vi "Master Setup Subpanel.vi"() -> ()   [LabVIEW 2017]
uses:
  Setup File Operations/File Operation with History Buttons.ctl
  Master Setup Export to Compressed Zip Folder.ctl
  Master Setup Import to Compressed Zip Folder.ctl
  Master Setup Open Backup Scheduler.ctl
  Setup File Operations/File Operation with History.ctl
  Master Setup States Enum.ctl
  <vilib>/Utility/miscctls.llb/LVRowAndColumnTypeDef.ctl
  Master Setup Pattern Enum.ctl
  <vilib>/Utility/config.llb/NI_LVConfig.lvlib
panel:
  in  "Backup Scheduler":T1
  in  "Tab Control":T2(tab)
  in  "Master Setup File List":i32(listbox)=-1
  out "Master Save Status":bool[](array[boolean])
  out "Master Open Status":bool[](array[boolean])
  out "Master Setup Titles":string[](array[string])=["0 - Channel Setup", "1 - PID Setup", "2 - Filter Setup", "3 - CAN Message Setup", "4 - CAN 1 Setup", "5 - CAN 2 Setup", "6 - Digital Inputs Setup", "7 - Digital Outputs Setup", "8 - Logging 1 Setup", "9 - Logging 2 Setup", "10 - Logging 3 Setup", "11 - Setpoint Setup", "12 - Test Series Setup", "13 - Graph Setup", "14 - System Configure", "15 - Header", "16 - Profile Manager", "17 - Post-Mortem Logging", "18 - High-Speed Data", "19 - Statistic Channel Setup", "20 - Ramp Channel Setup", "21 - ETAS INCA Channel Setup", "22 - ETC ECCS Transducer Setup", "23 - ETC ECCS Test Setup", "24 - AVL AK Smoke Meter Setup", "25 - Triggers Setup", "26 - Alarm Limits Setup", "27 - YKWT1 Measurement", "28 - YKWT1 Instrument", "29 - Auto File Settings", "30 - Playback File Setting", "31 - UUT Constants", "32 - UPS Setup", "33 - Differential Channel Setup", "34 - Integral Channel Setup", "35 - Signal Channel Setup", "36 - Calibration Setup", "37 - BNC Setup", "38 - ASAP3 Setup", "39 - Chassis Force Calculations", "40 - Chassis Teststand Losses", "41 - Chassis Vehicle Losses", "42 - Formula Channels", "43 - ASAP3 Map Coords Setup", "44 - Digital Controls Setup", "45 - Push Buttons Setup", "46 - Sliders Setup", "47 - Analog Inline Filter Setup", "48 - Email Setup", "49 - Timer Setup", "50 - Unit Conversion Setup", "51 - Visible Channels", "52 - Main Display Setup", "53 - Message Display Setup", "54 - Input Display Setup", "55 - Unico Parameter Downloads", "56 - Flow Meter Setup", "57 - Channel Zero Offset", "58 - YKWT2 Measurement", "59 - YKWT2 Instrument", "60 - CAN 3 Setup", "61 - CAS Setup", "62 - Accumulation Channel Setup", "63 - Valvetrain Dynamics Setup", "64 - CCP Setup", "65 - System Log Setup", "66 - Throttle Controller", "67 - RE Shifter", "68 - Main Display"]
  out "File Error":bool[](array[boolean])
  out "Convert Error":bool[](array[boolean])
  out "RT Update Error":bool[](array[boolean])
  in  "Refresh":bool
  in  "Master Open":bool
  in  "Master Save":bool
  in  "Master Exit":bool
  out "Login User":string
  out "Progress":i32(slide) scale=0.0..73.0
  out "File Path":path
  out "Last Time Saved":timestamp
  out "Master Open Indicator":bool
  out "Master Save Indicator":bool
  in  "WinZIP Import":T3
  in  "WinZIP Export":T4
  in  "File Operations with History Buttons":T5
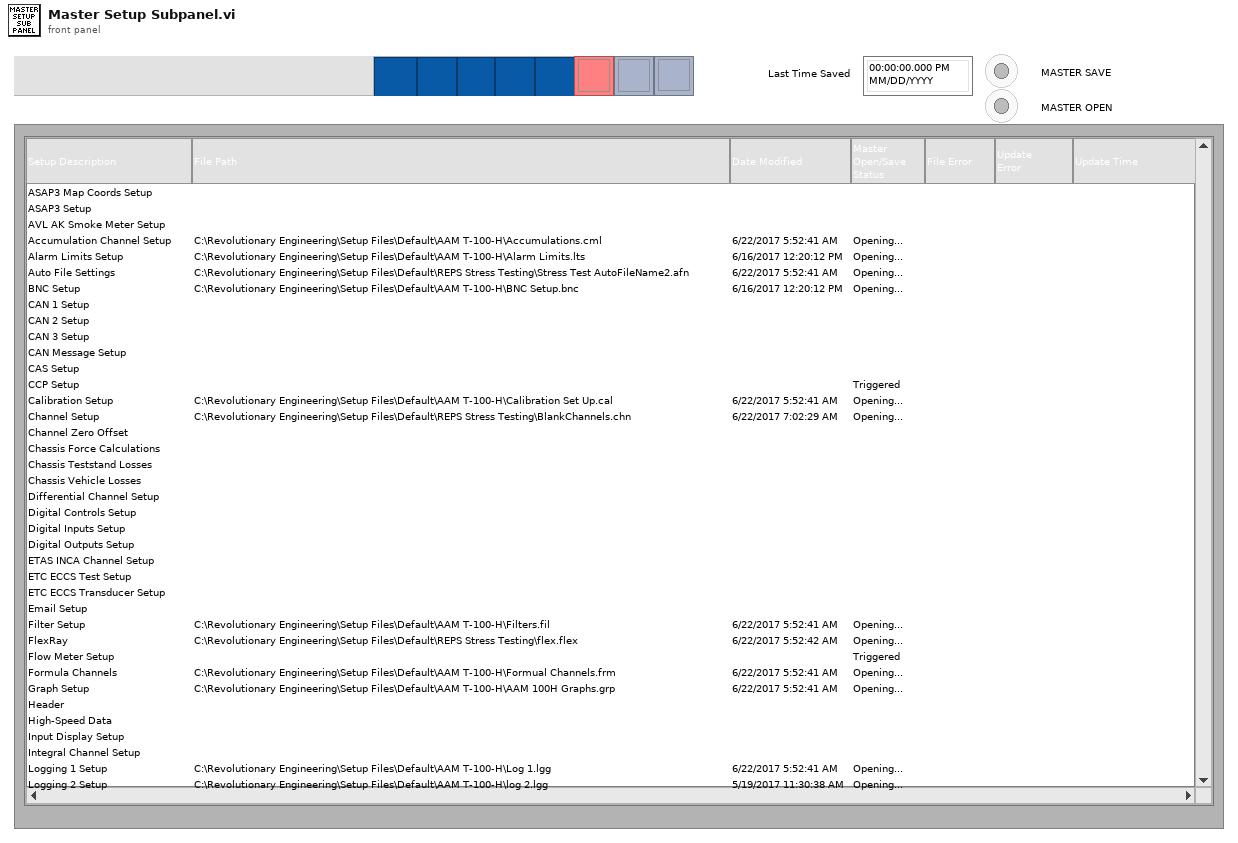
[diagram p1: front panel]
types:
  T1 = typedef "Master Setup Open Backup Scheduler.ctl" = bool
  T2 = enum32{"Master Setup List", "Master Setup Status", "File Update Event Log "}
  T3 = typedef "Master Setup Import to Compressed Zip Folder.ctl" = bool
  T4 = typedef "Master Setup Export to Compressed Zip Folder.ctl" = bool
  T5 = typedef "File Operation with History Buttons.ctl" = cluster{"New":bool, "Browse - Open":bool, "Save":bool, "Save As":bool, "Recent Files - Open":bool}
  T6 = typedef "Master Setup States Enum.ctl" = enum16{"Initialize", "Update Display", "Poll", "Prompt to Save", "Master Save", "Master Open", "Open Recent Dialog", "Open Normal Dialog", "Open Selected Master File", "WINZIP Export", "WINZIP Import", "WINZIP Auto Backup", "Exit"}
  T7 = typedef "File Operation with History.ctl" = cluster{"Operator New":bool, "Operator Open":bool, "Operator Save":bool, "Operator Save As":bool, "Master Open":bool, "Master Save":bool, "Shortcut Open (From Menu)":bool, "Shortcut Open (From Button)":bool}
  T8 = cluster{"Sorted Titles Indices":i32[], "Sorted Titles":string[], "Master Setup Path":path, "Master Setup Table":string[][], "First Run":bool, "Master Pattern":string, "Master Pattern Label":string, "Skip Save Prompt?":bool}
  T9 = typedef "LVRowAndColumnTypeDef.ctl" = cluster{"Row":i32, "Column":i32}
  T10 = enum16{"Read String Queue", "Write String Queue", "Read U16 Queue", "Write U16 Queue"}
  T11 = enum32{"Invalid", "Standard", "Closed", "Hidden", "Minimized", "Maximized"}
  T12 = enum16{"Get Master Open Status", "Get Master Save Status"}
  T13 = enum16{"open", "replace", "create", "open or create", "replace or create", "replace or create with confirmation"}
  T14 = typedef "PC_INI_Data__TypeDef.ctl" = cluster{"REPS Version":T15, "System Configuration":T16, "OPC PLC Write":string, "OPC PLC Read":string, "Modbus Info":string, "INCA Configuration":cluster{"IP":string, "Port":i32, "Protocol Version":i32}, "ECCS Setup":cluster{"Enable":bool, "IP":string, "TCP Port":u16, "UDP Port":u16, "Engine ODBC Name":string, "Fuel ODBC Name":string}, "Encoder Configuration":cluster{"Encoder1PPR":i32, "Encoder1Interval1":i32, "Encoder1Interval2":i32, "Roll Diameter(Feet)":i32, "Encoder2PPR":i32, "Encoder3PPR":i32, "Encoder4PPR":i32, "Encoder5PPR":i32, "Encoder2Interval1":i32, "Encoder2Interval2":i32, "Encoder3Interval1":i32, "Encoder3Interval2":i32}, "Pickup1 Configuration":cluster{"PickupPPR":i32, "PickupInterval1":i32, "PickupInterval2":i32}, "Pickup2 Configuration":cluster{"PickupPPR":i32, "PickupInterval1":i32, "PickupInterval2":i32}, "Pickup3 Configuration":cluster{"PickupPPR":i32, "PickupInterval1":i32, "PickupInterval2":i32}, "Shifter Configuration":cluster{"RE Shifter Enable":bool, "Shifter IP Address":string, "Shifter Port":u16}, "Misc Configuration":T17, "Logging Configuration":T18}
  T15 = typedef "REPS Version.ctl" = cluster{"Version":string}
  T16 = typedef "System Configuration.ctl" = cluster{"Cell":string, "DualMotorSet":bool, "Hardware Setup Array":bool[], "Host IP":string, "Remote IP 1":string, "Remote IP 2":string, "Remote IP 3":string, "Remote Enable 1":bool, "Remote Enable 2":bool, "Remote Enable 3":bool, "Company Name":string, "Company Info":string, "Number Of Modbus":i32, "Setup Files Path":path, "Master File Path":path, "Master Setup Titles":string[], "Encoder1PPR":i32, "Encoder1Interval1":i32, "Encoder1Interval2":i32, "Display File Error Status?":bool[], "Update to RT Delay":u32, "Formula Rate (Hz)":u32, "Custom Screen (Left) Path":path, "Custom Screen (Right) Path":path}
  T17 = typedef "Misc Configuration.ctl" = cluster{"Show PM Logging Indicator":bool}
  T18 = typedef "Logging Configuration.ctl" = cluster{"MaxLogFileSize":T19, "MaxNumofLogChannels":T19, "MaxNumofPMLogChannels":T19, "SkipPMDialog":i32}
  T19 = typedef "Framed Numeric 6 digit 20 point.ctl" = dbl
  T20 = typedef "NI_LVConfig.lvlib/Config Data RefNum.ctl" = refnum<k1>
  T21 = typedef "Master Setup Pattern Enum.ctl" = i32
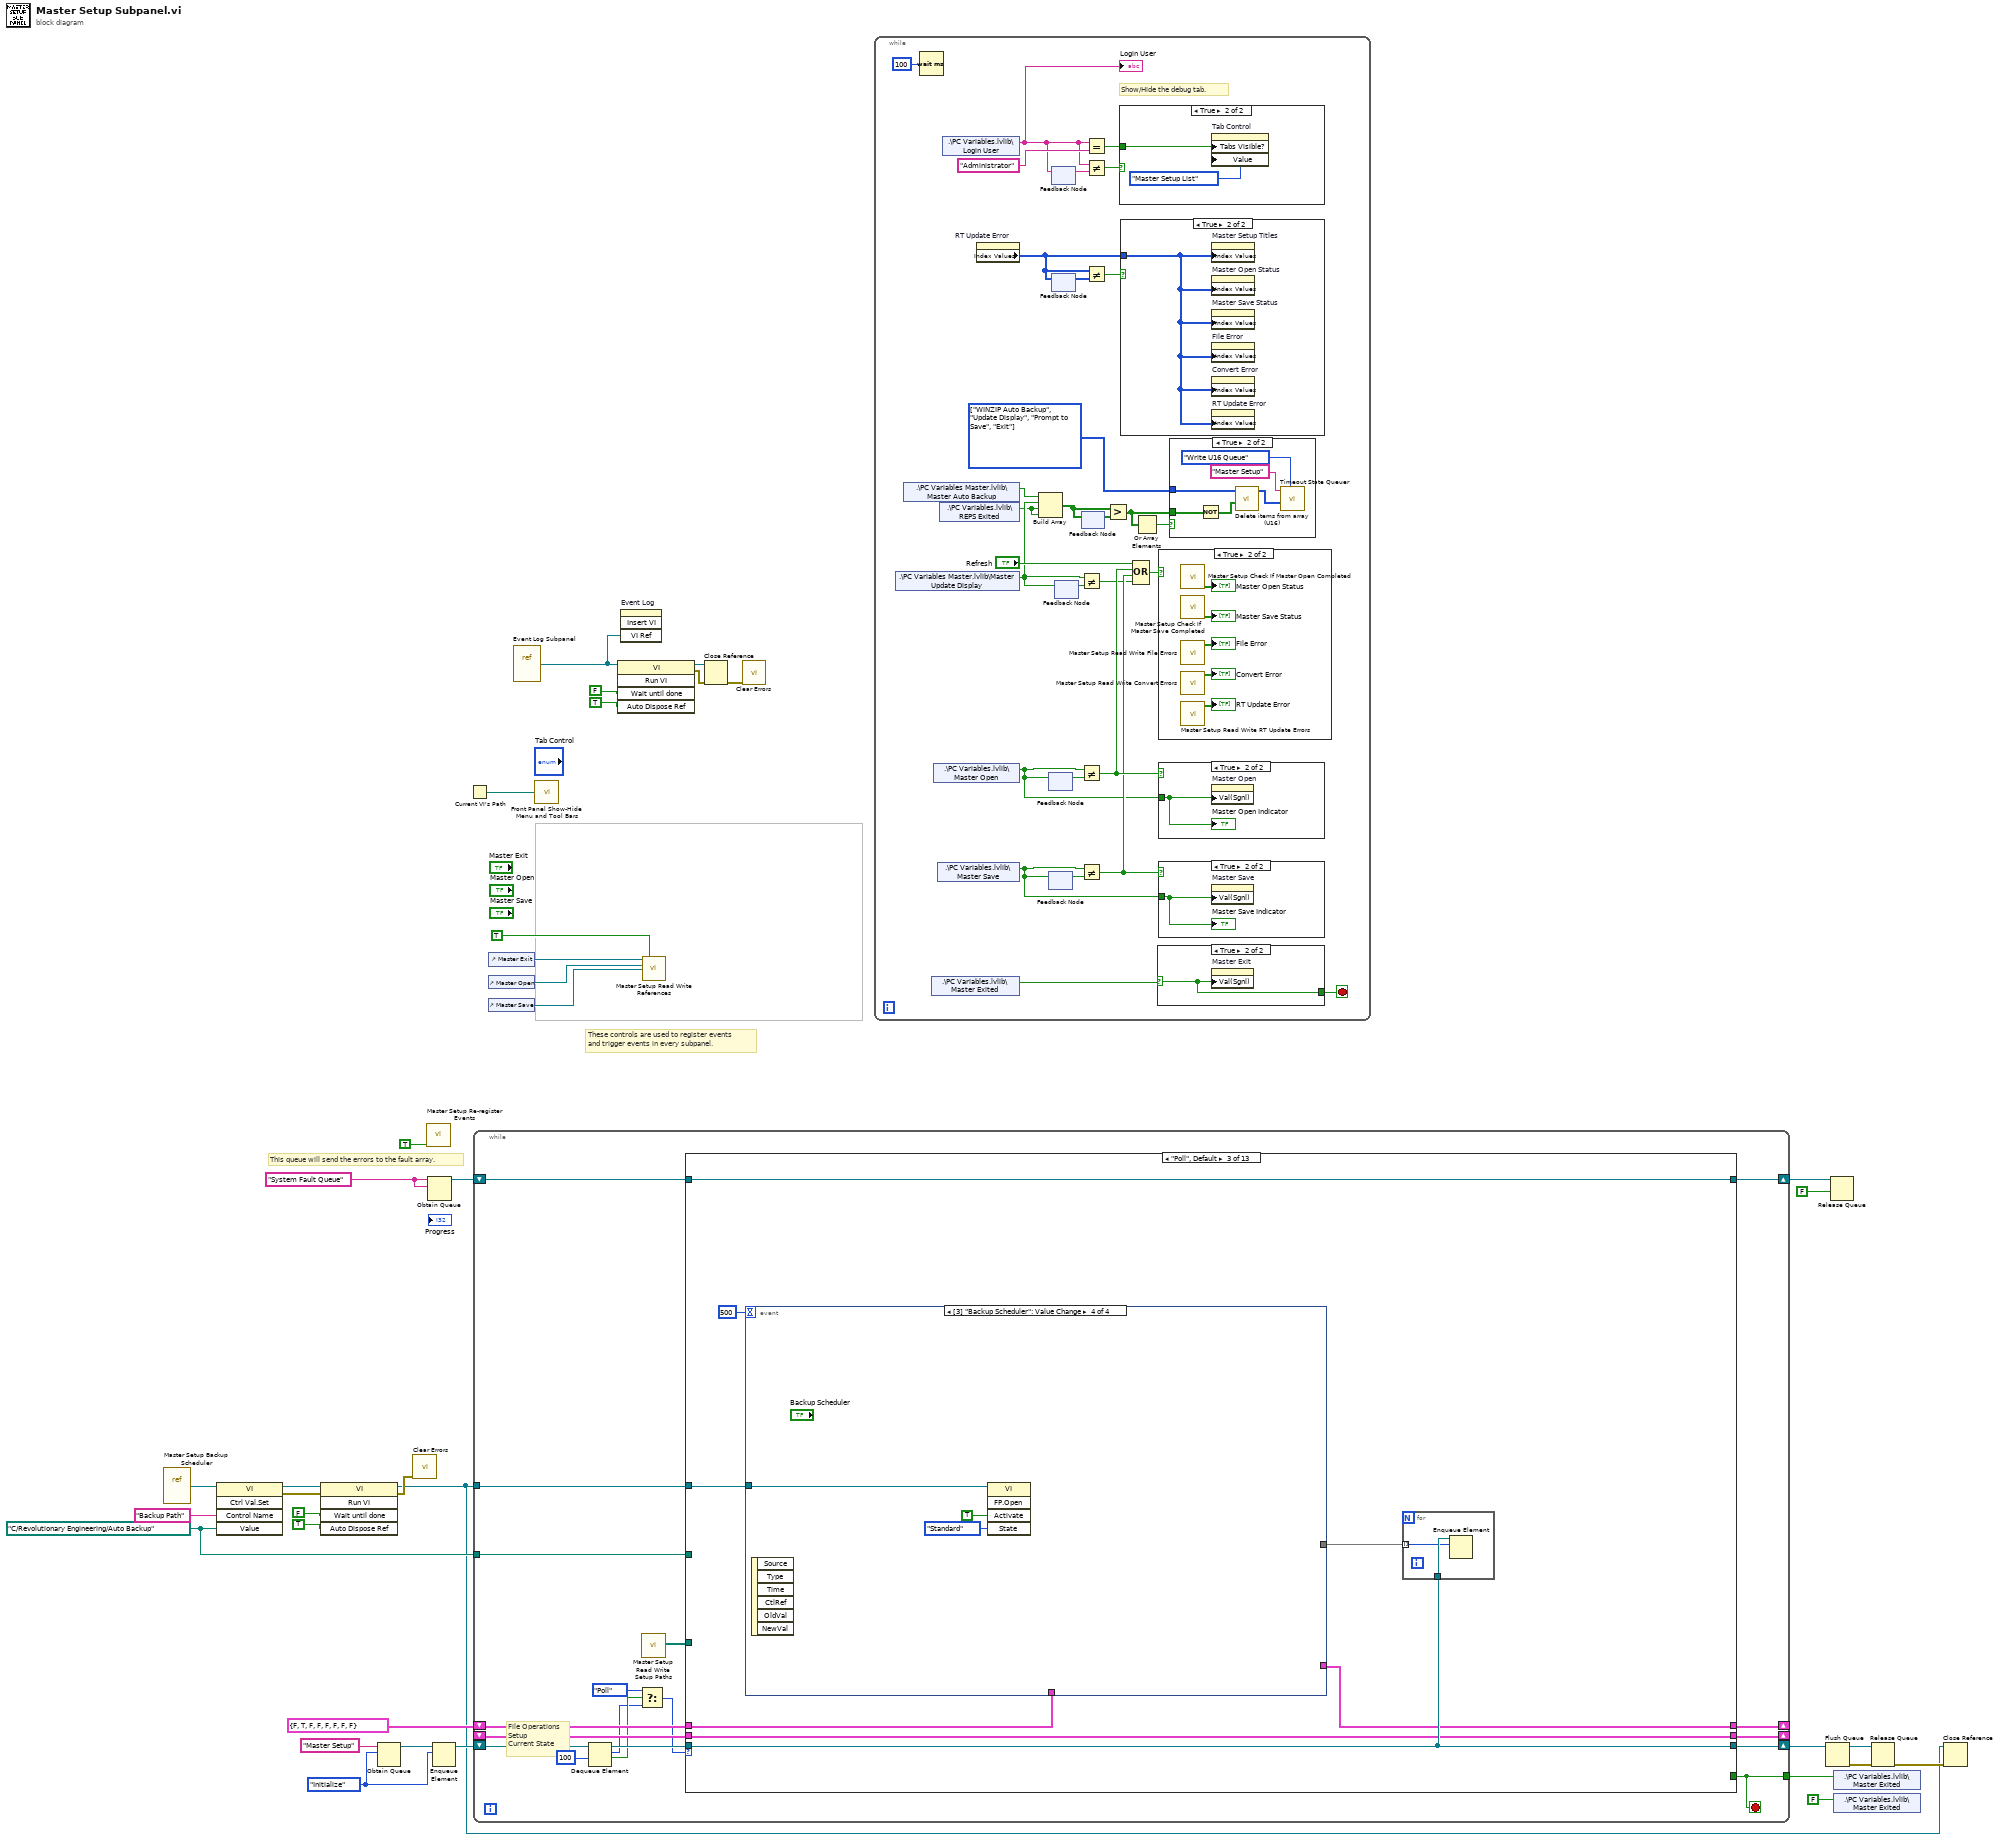
[diagram p0: block diagram]
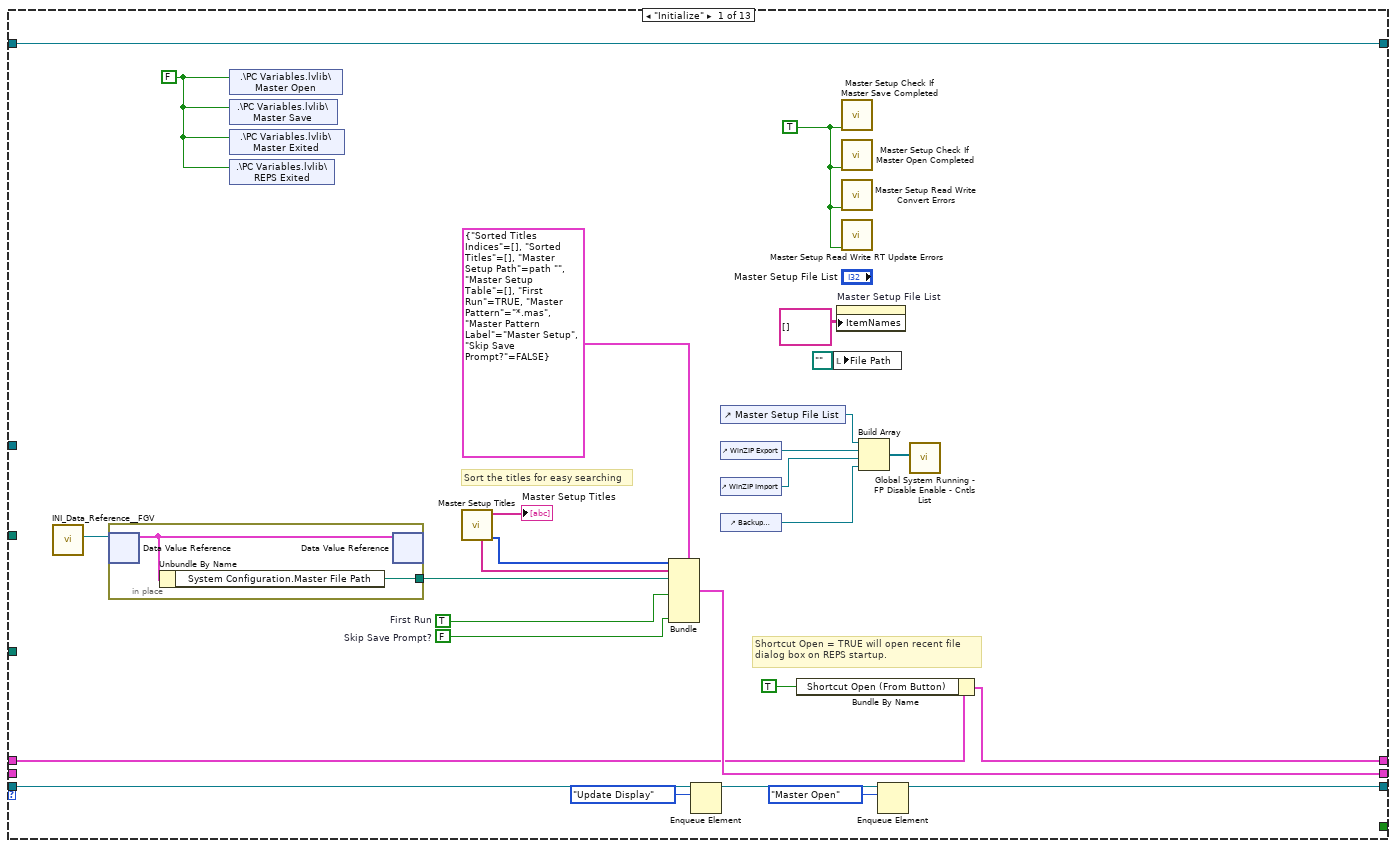
[diagram p9: hidden frame]
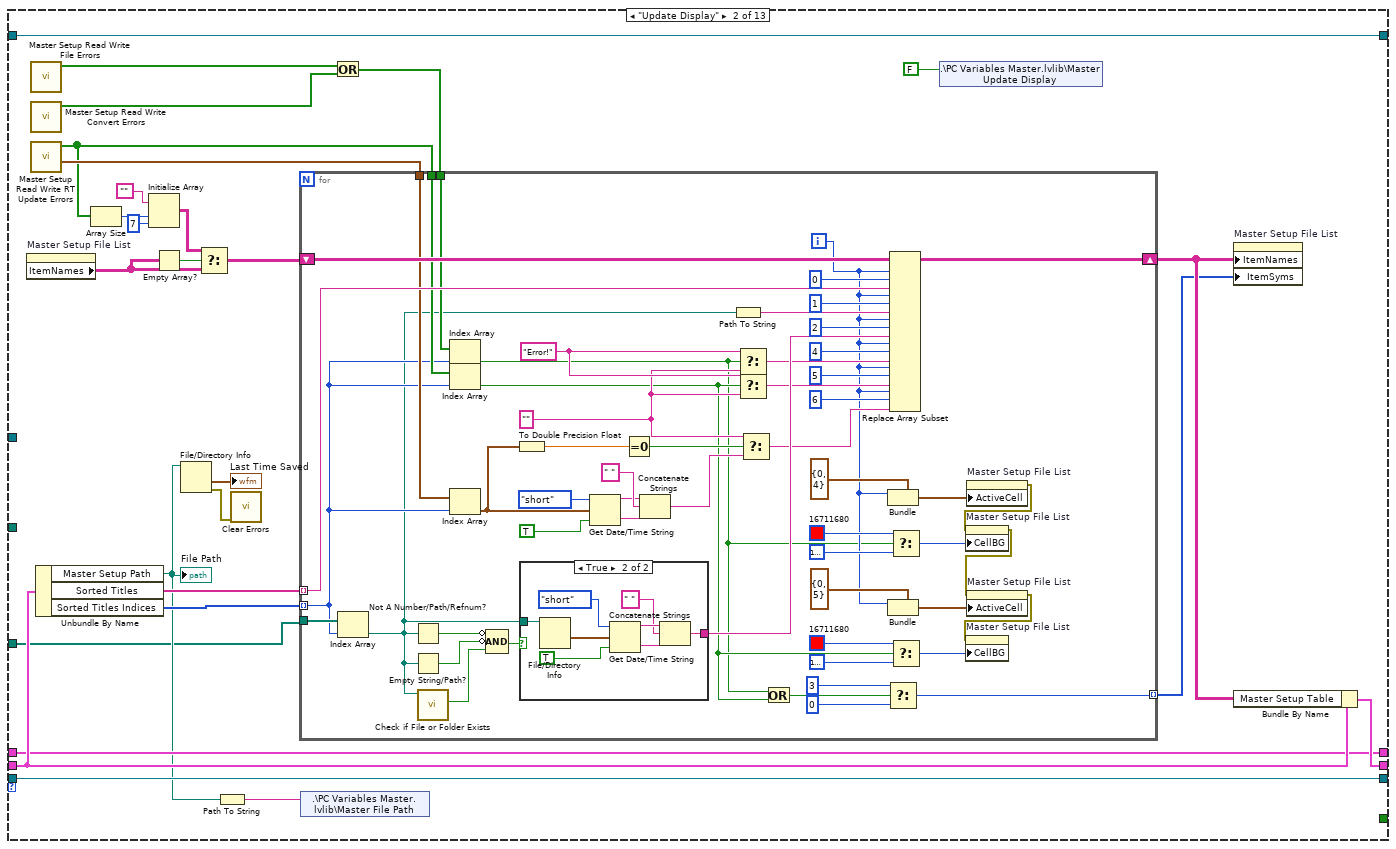
[diagram p10: hidden frame]
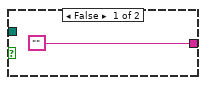
[diagram p11: hidden frame]
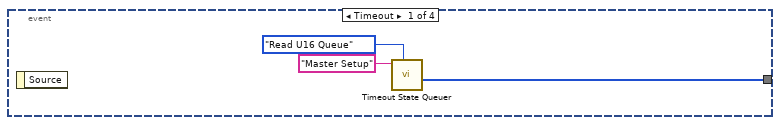
[diagram p12: hidden frame]
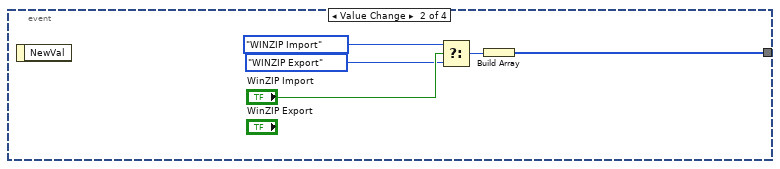
[diagram p13: hidden frame]
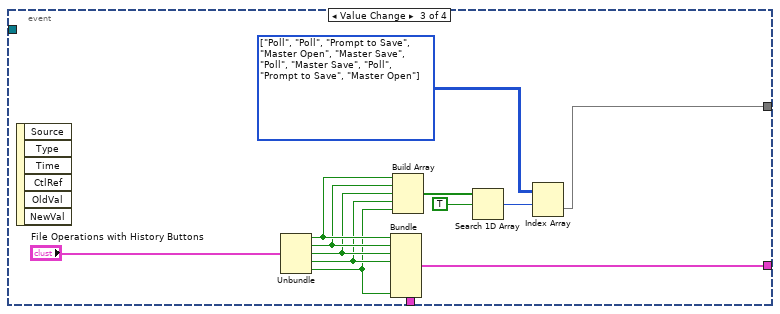
[diagram p14: hidden frame]
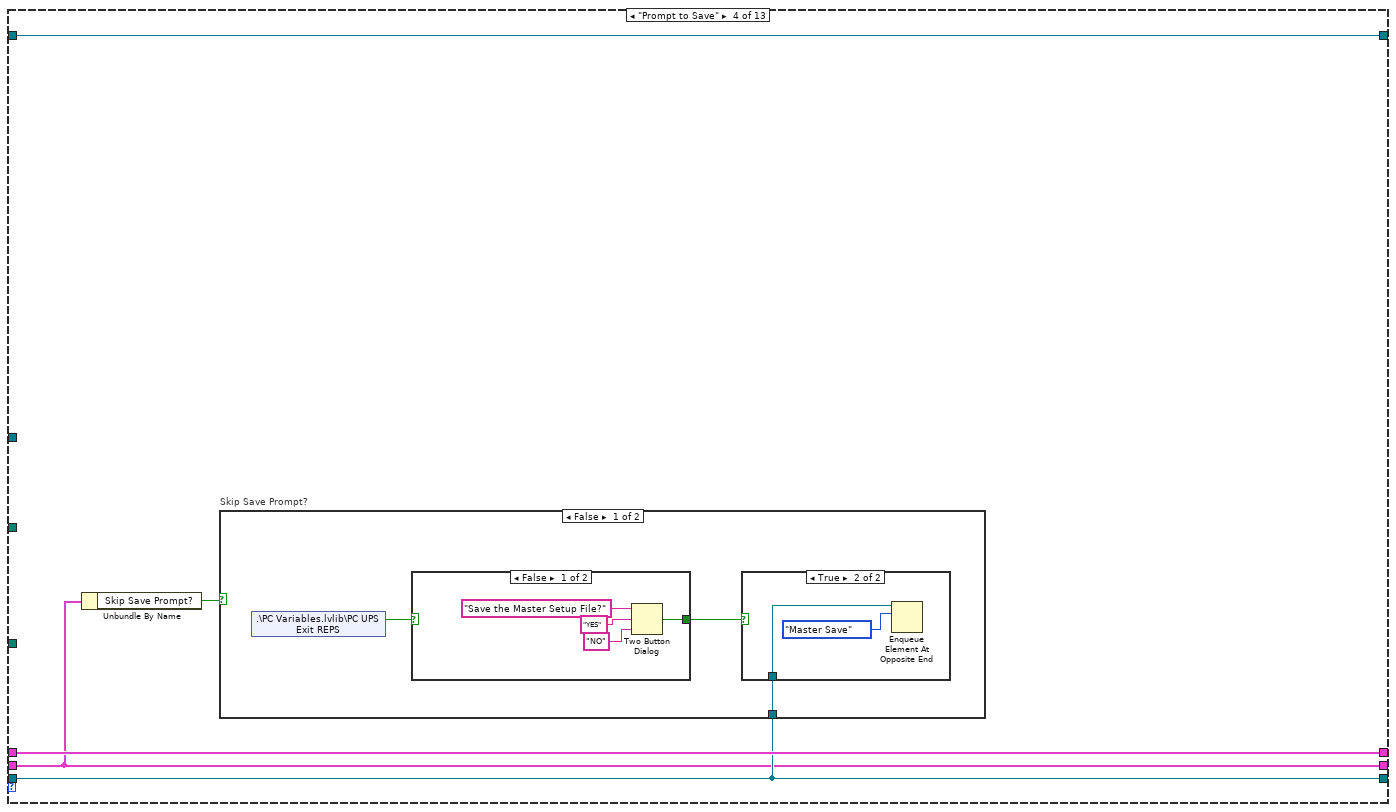
[diagram p15: hidden frame]
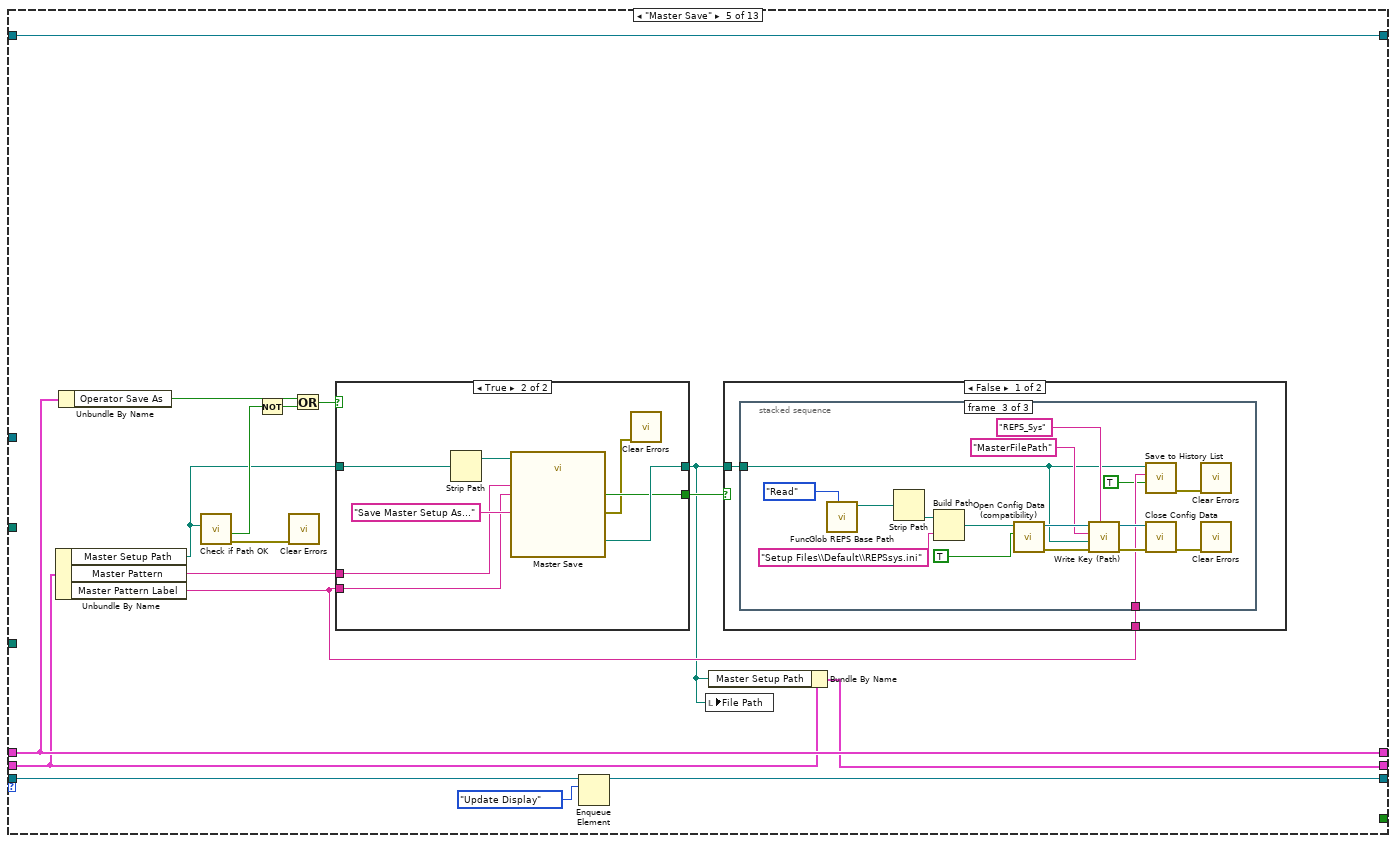
[diagram p19: hidden frame]
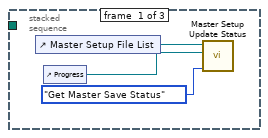
[diagram p20: hidden frame]
diagram:
  w5 = path "C:/Revolutionary Engineering/Auto Backup"
  w13 = Master_Setup_States_Enum."Initialize" ("States")
  w24 = "System Fault Queue" ("name (unnamed)")
  # "These controls are used to register events \nand trigger events in every subpanel."
  # "This queue will send the errors to the fault array."
  n1 = vi-ref "Master Setup Backup Scheduler.vi"() -> (w11:refnum<vi>)
  n2 = invoke class="VI" method="Ctrl Val.Set"(reference=w11, "Control Name"="Backup Path", "Value"=w5) -> (reference out=w8:refnum<vi>, error out=w9:errorcluster)  [unwired: 2 in, 3 out]
  n3 = invoke class="VI" method="Run VI"(reference=w8, error in=w9, "Wait until done"=FALSE ("Wait Until Done"), "Auto Dispose Ref"=TRUE ("Auto Dispose Reference")) -> (reference out=w3:refnum<vi>, error out=w12:errorcluster)  [unwired: 1 in, 3 out]
  n4 = Obtain Queue(name (unnamed)="Master Setup", element data type=w13) -> (queue out=w15:refnum<queue>)  [unwired: 3 in, 2 out]
  n5 = call <vilib>:"Clear Errors.vi"("error in (no error)"=w12) -> ()  [unwired: 5 in, 2 out]
  n6 = call "Master Setup Re-register Events.vi"("Master/Channel Subpanel Restarted"=TRUE) -> ()  [unwired: 10 in, 1 out]
  n7 = Obtain Queue(name (unnamed)=w24, element data type=w24) -> (queue out=w27:refnum<queue>)  [unwired: 3 in, 2 out]
  n8 = Enqueue Element(queue=w15, element=w13) -> (queue out=w14:refnum<queue>)  [unwired: 2 in, 2 out]
  n9 = Current VI's Path() -> (path=w22:path)
  n10 = while {
    shift-right: [w52] -> w32
    shift-left: w14 -> [w44]
    shift-right: [w51] -> _
    shift-left: _ -> [w54]
    shift-right: [w49] -> _
    shift-left: T7 {"Operator New"=FALSE, "Operator Open"=TRUE, "Operator Save"=FALSE, "Operator Save As"=FALSE, "Master Open"=FALSE, "Master Save"=FALSE, "Shortcut Open (From Menu)"=FALSE, "Shortcut Open (From Button)"=FALSE} ("File Operation (in)") -> [w48]
    tunnel: [w47] -> w1
    shift-right: [w45] -> w26
    shift-left: w27 -> [w46]
    tunnel: w5 -> [w38]
    tunnel: w3 -> [w37]
    stop <- w47 stop-if-true
    # "File Operations\nSetup\nCurrent State"
    n11 = Dequeue Element(queue=w44, timeout in ms (-1)=100) -> (queue out=w53:refnum<queue>, element=w42:T6, timed out?=w43:bool)  [unwired: 1 in, 1 out]
    n12 = Select(t=Master_Setup_States_Enum."Poll", s=w43, f=w42) -> (s? t:f=w40:T6)
    n13 = call "Master Setup Read Write Setup Paths.vi"() -> ("New Setup Paths"=w39:path[])  [unwired: 7 in, 4 out]
    n14 = case shown="\"Poll\", Default" w40 {
      tunnel: w54 -> [_ w95 w176 w210 w226 w283 w393 w439 w471 w494 w509 w533 w555]
      tunnel: w53 -> [w68 w110 w181 w211 w231 w285 w389 w442 w480 w495 w511 w549 w554]
      tunnel: [w75 w110 w181 w211 w230 w288 w388 w441 w480 w495 w505 w549 w554] -> w52
      tunnel: [w81 w107 w176 w210 w225 w284 w392 w438 w472 w494 w508 w533 w555] -> w51
      tunnel: [w64 w94 w179 w212 w227 w286 w399 w443 w479 w496 w512 w548 w556] -> w49
      tunnel: w48 -> [w65 w94 w180 w212 w227 w287 w399 w443 w479 w496 w512 w548 w556]
      tunnel: [_ _ _ _ _ _ _ _ _ _ _ _ TRUE] -> w47
      tunnel: w46 -> [w73 w90 w177 w213 w240 w289 w398 w450 w478 w490 w502 w547 w557]
      tunnel: [w73 w90 w177 w213 w240 w289 w398 w450 w478 w490 w502 w547 w557] -> w45
      tunnel: w39 -> [_ w86 _ _ _ _ _ _ _ w489 w500 w532 _]
      tunnel: w38 -> [_ _ _ _ _ _ _ _ _ _ _ w531 _]
      tunnel: w37 -> [_ _ w175 _ _ _ _ _ _ _ _ _ _]
      frame "Initialize" {
        w62 = FALSE  # Skip Save Prompt?
        w71 = FALSE ("Master Open")
        w74 = TRUE ("Reset")
        w66 = TRUE  # First Run
        # "Shortcut Open = TRUE will open recent file\ndialog box on REPS startup."
        # "Sort the titles for easy searching"
        n15 = call "INI_Data_Reference__FGV.vi"() -> (".ini Data Value Reference (out)"=w56:refnum<data-value>)  [unwired: 11 in]
        n16 = in-place {
          in-place-border: [w82] -> w55
          n17 = in-place-dvr #1(w56) -> (w83:T14)  [unwired: 1 out]
          n18 = Unbundle By Name(w83) -> ("System Configuration.Master File Path"=w82:path)
          n19 = in-place-dvr #1(w83) -> ()  [unwired: 2 out]
        }
        n20 = shared-variable ".\\PC Variables.lvlib\\Master Open"(w71) -> ()  [unwired: 1 in, 1 out]
        n21 = shared-variable ".\\PC Variables.lvlib\\Master Save"(w71) -> ()  [unwired: 1 in, 1 out]
        n22 = shared-variable ".\\PC Variables.lvlib\\Master Exited"(w71) -> ()  [unwired: 1 in, 1 out]
        n23 = shared-variable ".\\PC Variables.lvlib\\REPS Exited"(w71) -> ()  [unwired: 1 in, 1 out]
        n24 = call "Master Setup Titles.vi"() -> ("Sorted Titles Indices"=w76:i32[], "Setup Description w/Numbers"=→"Master Setup Titles":string[], "Sorted Setup Description"=w77:string[])  [unwired: 6 in, 3 out]
        n25 = Bundle(cluster=T8 {"Sorted Titles Indices"=[], "Sorted Titles"=[], "Master Setup Path"=path "", "Master Setup Table"=[], "First Run"=TRUE, "Master Pattern"="*.mas", "Master Pattern Label"="Master Setup", "Skip Save Prompt?"=FALSE}, "Sorted Titles Indices"=w76, "Sorted Titles"=w77, "Master Setup Path"=w55, "First Run"=w66, "Skip Save Prompt?"=w62) -> (w81:T8)  [unwired: 3 in]
        n26 = Enqueue Element(queue=w68, element=Master_Setup_States_Enum."Update Display") -> (queue out=w67:refnum<queue>)  [unwired: 2 in, 2 out]
        n27 = control-ref of="Master Setup File List"() -> (w60:refnum<vi>)
        n28 = control-ref of="WinZIP Export"() -> (w59:refnum<vi>)
        n29 = control-ref of="WinZIP Import"() -> (w58:refnum<vi>)
        n30 = control-ref of="Backup Scheduler"() -> (w57:refnum<vi>)
        n31 = Bundle By Name(cluster=w65, "Shortcut Open (From Button)"=TRUE) -> (w64:T7)
        n32 = local write "File Path"(path "" ("File Path")) -> ()
        n33 = property on="Master Setup File List" class="MCListbox (strict)"("ItemNames"=string[][] [] ("Item Names")) -> ()  [unwired: 2 in, 2 out]
        n34 = call "Master Setup Check If Master Save Completed.vi"("Reset"=w74) -> ()  [unwired: 6 in, 5 out]
        n35 = call "Master Setup Check If Master Open Completed.vi"("Reset"=w74) -> ()  [unwired: 6 in, 5 out]
        n36 = call "Master Setup Read Write Convert Errors.vi"("Reset"=w74) -> ()  [unwired: 9 in, 2 out]
        n37 = call "Master Setup Read Write RT Update Errors.vi"("Reset"=w74) -> ()  [unwired: 8 in, 3 out]
        n38 = Build Array(w60, w59, w58, w57) -> (w61:refnum<vi>[])
        n39 = Enqueue Element(queue=w67, element=Master_Setup_States_Enum."Master Open") -> (queue out=w75:refnum<queue>)  [unwired: 2 in, 2 out]
        n40 = call "Global System Running - FP Disable Enable - Cntls List.vi"("Cntls Should NOT be disabled In[]"=w61) -> ()  [unwired: 8 in, 3 out]
      }
      frame "Update Display" {
        n41 = property on="Master Setup File List" class="MCListbox (strict)"() -> ("ItemNames"=w103:string[][])  [unwired: 2 in, 2 out]
        n42 = call "Master Setup Read Write File Errors.vi"() -> ("File Error (out)"=w93:bool[])  [unwired: 10 in, 1 out]
        n43 = call "Master Setup Read Write Convert Errors.vi"() -> ("Convert Error (out)"=w92:bool[])  [unwired: 10 in, 1 out]
        n44 = call "Master Setup Read Write RT Update Errors.vi"() -> ("Update Timestamp"=w97:timestamp[], "Real-Time Update Status (out)"=w96:bool[])  [unwired: 9 in, 1 out]
        n45 = Unbundle By Name(w95) -> ("Master Setup Path"=w87:path, "Sorted Titles"=w108:string[], "Sorted Titles Indices"=w109:i32[])
        "File Path" <- w87
        n46 = Array Size(array=w96) -> (size(s)=w102:i32)
        n47 = Initialize Array("", w102, 7 ("dimension size")) -> (w99:string[][])
        n48 = Empty Array?(array=w103) -> (empty?=w105:bool)
        n49 = File/Directory Info(path=w87) -> (last mod=→"Last Time Saved":timestamp, error out=w88:errorcluster)  [unwired: 1 in, 5 out]
        n50 = Select(t=w99, s=w105, f=w103) -> (s? t:f=w104:string[][])
        n51 = Path To String(path=w87) -> (string=w84:string)
        n52 = call <vilib>:"Clear Errors.vi"("error in (no error)"=w88) -> ()  [unwired: 5 in, 2 out]
        n53 = shared-variable ".\\PC Variables Master.lvlib\\Master File Path"(w84) -> ()  [unwired: 1 in, 1 out]
        n54 = Or(x=w93, y=w92) -> (x .or. y?=w91:bool[])
        n55 = for {
          tunnel: w86 -> [w162]
          tunnel: w109 -> [w123] mode=indexing
          tunnel: w108 -> [w158] mode=indexing
          tunnel: w91 -> [w124]
          tunnel: w96 -> [w125]
          shift-right: [w159] -> w106
          shift-left: w104 -> [w160]
          tunnel: [w143] -> w98 mode=indexing
          tunnel: w97 -> [w127]
          i -> [w116]
          w128 = ""
          w130 = "Error!" ("Setup Description")
          n56 = Index Array(array=w162, index=w123) -> (element=w111:path)
          n57 = Not A Number/Path/Refnum?(number/path/refnum=w111) -> (NaN/Path/Refnum?=w163:bool)
          n58 = Empty String/Path?(string/path=w111) -> (empty?=w165:bool)
          n59 = call <vilib>:"Check if File or Folder Exists.vi"("path"=w111) -> ("file or folder exists?"=w164:bool)  [unwired: 8 in, 2 out]
          n60 = Index Array(array=w124, index=w123) -> (element=w114:bool)
          n61 = Index Array(array=w125, index=w123) -> (element=w115:bool)
          n62 = Index Array(array=w127, index=w123) -> (element=w126:timestamp)
          n63 = Compound Arithmetic op=AND(invert w163, invert w165, w164) -> (w161:bool)
          n64 = To Double Precision Float(number=w126) -> (double precision float=w137:dbl)
          n65 = case shown="True" w161 {
            tunnel: ["" w174] -> w152
            tunnel: w111 -> [_ w173]
            frame False {
            }
            frame True {
              n66 = File/Directory Info(path=w173) -> (last mod=w172:timestamp)  [unwired: 1 in, 6 out]
              n67 = Get Date/Time String(date format (0)=enum16{"short", "long", "abbreviated"}."short", seconds (now)=w172, want seconds? (F)=TRUE) -> (date string=w170:string, time string=w169:string)
              n68 = Concatenate Strings(w170, " " ("string"), w169) -> (w174:string)
            }
          }
          n69 = Get Date/Time String(date format (0)=enum16{"short", "long", "abbreviated"}."short", seconds (now)=w126, want seconds? (F)=TRUE) -> (date string=w139:string, time string=w140:string)
          n70 = Equal To 0?(x=w137) -> (x = 0?=w136:bool)
          n71 = Concatenate Strings(w139, " " ("string"), w140) -> (w135:string)
          n72 = Path To String(path=w111) -> (string=w153:string)
          n73 = Select(t=w130, s=w114, f=w128) -> (s? t:f=w131:string)
          n74 = Select(t=w130, s=w115, f=w128) -> (s? t:f=w129:string)
          n75 = Select(t=w128, s=w136, f=w135) -> (s? t:f=w134:string)
          n76 = Or(x=w114, y=w115) -> (x .or. y?=w113:bool)
          n77 = Bundle(cluster=T9 {"Row"=0, "Column"=4} ("Active Cell:Active Cell"), "Row"=w116) -> (w147:T9)  [unwired: 1 in]
          n78 = Bundle(cluster=T9 {"Row"=0, "Column"=5} ("Active Cell:Active Cell"), "Row"=w116) -> (w121:T9)  [unwired: 1 in]
          n79 = Select(t=3 ("Column"), s=w113, f=0 ("Column")) -> (s? t:f=w143:i32)
          n80 = Replace Array Subset(array=w160, new element #1=w158, index (row) #1=w116, index (col) #1=0 ("disabled index (col)"), new element #2=w153, index (row) #2=w116, index (col) #2=1 ("disabled index (col)"), new element #3=w152, index (row) #3=w116, index (col) #3=2 ("disabled index (col)"), new element #4=w131, index (row) #4=w116, index (col) #4=4 ("disabled index (col)"), new element #5=w129, index (row) #5=w116, index (col) #5=5 ("disabled index (col)"), new element #6=w134, index (row) #6=w116, index (col) #6=6 ("disabled index (col)")) -> (w159:string[][])
          n81 = Select(t=u32 16711680, s=w114, f=u32 16777226) -> (s? t:f=w146:u32)
          n82 = Select(t=u32 16711680, s=w115, f=u32 16777226) -> (s? t:f=w122:u32)
          n83 = property on="Master Setup File List" class="MCListbox (strict)"("ActiveCell"=w147) -> (error out=w150:errorcluster)  [unwired: 2 in, 1 out]
          n84 = property on="Master Setup File List" class="MCListbox (strict)"(error in=w150, "CellBG"=w146) -> (error out=w112:errorcluster)  [unwired: 1 in, 1 out]
          n85 = property on="Master Setup File List" class="MCListbox (strict)"(error in=w112, "ActiveCell"=w121) -> (error out=w118:errorcluster)  [unwired: 1 in, 1 out]
          n86 = property on="Master Setup File List" class="MCListbox (strict)"(error in=w118, "CellBG"=w122) -> ()  [unwired: 1 in, 2 out]
        }
        n87 = shared-variable ".\\PC Variables Master.lvlib\\Master Update Display"(FALSE ("Master Update Display")) -> ()  [unwired: 1 in, 1 out]
        n88 = property on="Master Setup File List" class="MCListbox (strict)"("ItemNames"=w106, "ItemSyms"=w98) -> ()  [unwired: 2 in, 2 out]
        n89 = Bundle By Name(cluster=w95, "Master Setup Table"=w106) -> (w107:T8)
      }
      frame "Poll", Default {
        n90 = event shown="[3] \"Backup Scheduler\": Value Change" {
          selector: _ -> [_ _ _ _]
          dyn-events: _ -> [_ _ _ _]
          timeout: 500 -> [_ _ _ _]
          tunnel: [w187 w190 w193 _] -> w182
          tunnel: w180 -> [_ _ w204 _]
          tunnel: [_ _ w203 _] -> w179
          tunnel: w175 -> [_ _ _ w206]
          event Timeout {
            n91 = event-data() -> ()  [unwired: 1 in, 1 out]
            n92 = call "Timeout State Queuer.vi"("Action"=T10."Read U16 Queue", "Name of queue"="Master Setup") -> ("Queued states (U16)"=w187:u16[])  [unwired: 8 in, 1 out]
          }
          event Value Change {
            n93 = event-data() -> ()  [unwired: 1 in, 1 out]
            n94 = Select(t=Master_Setup_States_Enum."WINZIP Import" ("States"), s="WinZIP Import", f=Master_Setup_States_Enum."WINZIP Export" ("States")) -> (s? t:f=w191:T6)
            n95 = Build Array(w191) -> (w190:T6[])
          }
          event Value Change {
            w194 = T6[][] [[enum."Poll", enum."Poll"], [enum."Prompt to Save", enum."Master Open"], [enum."Master Save", enum."Poll"], [enum."Master Save", enum."Poll"], [enum."Prompt to Save", enum."Master Open"]] items=["Initialize", "Update Display", "Poll", "Prompt to Save", "Master Save", "Master Open", "Open Recent Dialog", "Open Normal Dialog", "Open Selected Master File", "WINZIP Export", "WINZIP Import", "WINZIP Auto Backup", "Exit"]
            n96 = event-data() -> ()  [unwired: 1 in, 6 out]
            n97 = Unbundle("File Operations with History Buttons") -> ("New"=w202:bool, "Browse - Open"=w201:bool, "Save"=w200:bool, "Save As"=w199:bool, "Recent Files - Open"=w198:bool)
            n98 = Bundle(cluster=w204, "Operator New"=w202, "Operator Open"=w201, "Operator Save"=w200, "Operator Save As"=w199, "Shortcut Open (From Button)"=w198) -> (w203:T7)  [unwired: 3 in]
            n99 = Build Array(w202, w201, w200, w199, w198) -> (w197:bool[])
            n100 = Search 1D Array(1D array=w197, element=TRUE) -> (index of element=w195:i32)  [unwired: 1 in]
            n101 = Index Array(array=w194, index (row)=w195) -> (element=w193:T6[])  [unwired: 1 in]
          }
          event Value Change {
            n102 = event-data() -> ()  [unwired: 1 in, 6 out]
            n103 = invoke class="VI" method="FP.Open"(reference=w206, "Activate"=TRUE ("Activate?"), "State"=T11."Standard") -> ()  [unwired: 2 in, 5 out]
          }
        }
        n104 = for {
          tunnel: w182 -> [w183] mode=indexing
          tunnel: w181 -> [w184]
          n105 = Enqueue Element(queue=w184, element=w183) -> ()  [unwired: 2 in, 3 out]
        }
      }
      frame "Prompt to Save" {
        n106 = Unbundle By Name(w210) -> ("Skip Save Prompt?"=w209:bool)
        n107 = case "Skip Save Prompt?" shown="False" w209 {
          tunnel: w211 -> [w215 _]
          frame False {
            n108 = shared-variable ".\\PC Variables.lvlib\\PC UPS Exit REPS"() -> (w214:bool)  [unwired: 1 in, 1 out]
            n109 = case shown="False" w214 {
              selector: w214 -> [_ w223]
              tunnel: [w221 w223] -> w216
              frame False {
                n110 = Two Button Dialog(message="Save the Master Setup File?", 1:"NO" ("F button name (\"Cancel\")"), 2:"YES" ("T button name (\"OK\")")) -> (T button?=w221:bool)
              }
              frame True {
              }
            }
            n111 = case shown="True" w216 {
              tunnel: w215 -> [_ w218]
              frame False {
              }
              frame True {
                n112 = Enqueue Element At Opposite End(queue=w218, element=Master_Setup_States_Enum."Master Save") -> ()  [unwired: 2 in, 3 out]
              }
            }
          }
          frame True {
            # "If true, skip the Save prompt."
          }
        }
      }
      frame "Master Save" {
        n113 = Unbundle By Name(w226) -> ("Master Setup Path"=w233:path, "Master Pattern"=w234:string, "Master Pattern Label"=w228:string)
        n114 = Unbundle By Name(w227) -> ("Operator Save As"=w238:bool)
        n115 = call "Check if Path OK.vi"("Path"=w233) -> ("error out"=w239:errorcluster, "Path OK"=w237:bool)  [unwired: 8 in, 1 out]
        n116 = Not(x=w237) -> (.not. x?=w235:bool)
        n117 = call <vilib>:"Clear Errors.vi"("error in (no error)"=w239) -> ()  [unwired: 5 in, 2 out]
        n118 = Or(x=w238, y=w235) -> (x .or. y?=w236:bool)
        n119 = case shown="True" w236 {
          tunnel: w234 -> [_ w280]
          tunnel: w228 -> [_ w278]
          tunnel: w233 -> [w274 w279]
          tunnel: [w274 w277] -> w224
          tunnel: [FALSE ("cancelled") w276] -> w232
          frame False {
          }
          frame True {
            n120 = Strip Path(path=w279) -> (stripped path=w282:path)  [unwired: 1 out]
            n121 = call "Master Save"("start path"=w282, "prompt"="Save Master Setup As...", "pattern (all files)"=w280, "pattern label"=w278) -> ("selected path"=w277:path, "cancelled"=w276:bool, "error out"=w275:errorcluster)  [unwired: 8 in, 1 out]
            n122 = call <vilib>:"Clear Errors.vi"("error in (no error)"=w275) -> ()  [unwired: 5 in, 2 out]
          }
        }
        n123 = Enqueue Element(queue=w231, element=Master_Setup_States_Enum."Update Display") -> (queue out=w230:refnum<queue>)  [unwired: 2 in, 2 out]
        n124 = local write "File Path"(w224) -> ()
        n125 = Bundle By Name(cluster=w226, "Master Setup Path"=w224) -> (w225:T8)
        n126 = case shown="False" w232 {
          tunnel: w224 -> [w242 _]
          tunnel: w228 -> [w241 _]
          frame False {
            n127 = stacked-sequence {
              tunnel: w242 -> [_ w249 w260]
              tunnel: w241 -> [_ _ w259]
              frame #0 {
                n128 = control-ref of="Master Setup File List"() -> (w243:refnum<vi>)
                n129 = control-ref of="Progress"() -> (w244:refnum<vi>)
                n130 = call "Master Setup Update Status.vi"("Function"=T12."Get Master Save Status", "Progress Bar Refnum"=w244, "Master Setup List Refnum"=w243) -> ()  [unwired: 5 in]
              }
              frame #1 {
                n131 = call "Master Setup Read Write Setup Paths.vi"() -> ("New Setup Paths"=w250:path[])  [unwired: 7 in, 4 out]
                n132 = Path To String(path=w250) -> (string=w247:string[])
                n133 = Open/Create/Replace File(file path (use dialog)=w249, operation (0:open)=T13."replace or create") -> (refnum out=w254:refnum<file>, error out=w251:errorcluster)  [unwired: 4 in, 1 out]
                n134 = To Variant(anything=w247) -> (Variant=w246:variant)
                n135 = Write to Binary File(file (use dialog)=w254, data=w246, error in=w251) -> (refnum out=w253:refnum<file>, error out=w252:errorcluster)  [unwired: 3 in, 1 out]
                n136 = Close File(refnum=w253, error in=w252) -> (error out=w248:errorcluster)  [unwired: 1 out]
                n137 = call <vilib>:"Clear Errors.vi"("error in (no error)"=w248) -> ()  [unwired: 5 in, 2 out]
              }
              frame #2 {
                n138 = call "FuncGlob REPS Base Path.vi"("Action"=enum16{"Read", "Write"}."Read") -> ("REPS Base Path"=w262:path)  [unwired: 10 in]
                n139 = Strip Path(path=w262) -> (stripped path=w271:path)  [unwired: 1 out]
                n140 = Build Path(base path=w271, name or relative path="Setup Files\\Default\\REPSsys.ini") -> (appended path=w269:path)
                n141 = call <vilib>:"Open Config Data (compatibility).vi"("create file if necessary (T)"=TRUE ("create file if necessary? (T)"), "configuration file path"=w269) -> ("error out"=w272:errorcluster, "refnum"=w267:T20)  [unwired: 7 in, 1 out]
                n142 = call <vilib>:"Write Key (Path).vi"("section"="REPS_Sys", "error in (no error)"=w272, "value"=w260, "key"="MasterFilePath", "refnum"=w267) -> ("error out"=w263:errorcluster, "refnum out"=w266:T20)  [unwired: 4 in, 1 out]
                n143 = call "Save to History List.vi"("Write to History File"=TRUE, "File pattern label"=w259, "File Path In"=w260) -> ("error out"=w257:errorcluster)  [unwired: 5 in, 3 out]
                n144 = call <vilib>:"Close Config Data.vi"("error in (no error)"=w263, "refnum"=w266) -> ("error out"=w261:errorcluster)  [unwired: 8 in, 1 out]
                n145 = call <vilib>:"Clear Errors.vi"("error in (no error)"=w257) -> ()  [unwired: 5 in, 2 out]
                n146 = call <vilib>:"Clear Errors.vi"("error in (no error)"=w261) -> ()  [unwired: 5 in, 2 out]
              }
            }
          }
          frame True {
          }
        }
      }
      frame "Master Open" {
        n147 = disable-structure shown="Disabled" {
          disable-tunnel: [w297 w383] -> w288
          disable-tunnel: w287 -> [w296 w378]
          disable-tunnel: [w295 w378] -> w286
          disable-tunnel: w285 -> [w293 w384]
          disable-tunnel: [w291 w377] -> w284
          disable-tunnel: w283 -> [w290 w377]
          frame Disabled {
            n148 = Unbundle By Name(w296) -> ("Shortcut Open (From Button)"=w299:bool)
            n149 = Unbundle By Name(w290) -> ("First Run"=w292:bool)
            n150 = case shown="False" w299 {
              tunnel: [w358 w369] -> w298
              tunnel: [w357 w371] -> w302
              tunnel: w290 -> [w356 w372]
              tunnel: [w355 _] -> w301
              tunnel: [w354 w368] -> w300
              tunnel: [_ w367] -> w294
              tunnel: w292 -> [_ w363]
              frame False {
                n151 = Unbundle By Name(w356) -> ("Master Setup Path"=w360:path, "Master Pattern"=w362:string, "Master Pattern Label"=w354:string)
                n152 = Strip Path(path=w360) -> (stripped path=w359:path)  [unwired: 1 out]
                n153 = call "File Dialog"("start path"=w359, "prompt"="Please Select a Master Setup File to Open...", "pattern (all files)"=w362, "pattern label"=w354) -> ("selected path"=w358:path, "cancelled"=w357:bool, "error out"=w355:errorcluster)  [unwired: 8 in, 1 out]
              }
              frame True {
                n154 = Unbundle By Name(w372) -> ("Master Pattern Label"=w368:string)
                n155 = Select(t="Exit REPS" ("Cancel Button String"), s=w363, f="") -> (s? t:f=w364:string)
                n156 = call "Prompt for Recent Files.vi"("File pattern label"=w368, "Cancel Button String"=w364) -> ("File to Open"=w370:string, "Cancelled"=w371:bool, "Browse for file"=w367:bool)  [unwired: 1 in]
                n157 = String To Path(string=w370) -> (path=w369:path)
              }
            }
            n158 = local write "File Path"(w298) -> ()
            n159 = call <vilib>:"Clear Errors.vi"("error in (no error)"=w301) -> ()  [unwired: 5 in, 2 out]
            n160 = case "Browse option selected in recent files dialog?" shown="False" w294 {
              tunnel: w302 -> [w312 _]
              tunnel: w300 -> [w311 _]
              tunnel: w298 -> [w310 _]
              tunnel: w290 -> [w309 w353]
              tunnel: w292 -> [w308 _]
              tunnel: [w307 w353] -> w291
              tunnel: w293 -> [w303 w351]
              tunnel: [w304 w350] -> w297
              tunnel: w296 -> [w306 w349]
              tunnel: [w306 w348] -> w295
              frame False {
                n161 = case "Get Recent Dialog Cancelled?" shown="False" w312 {
                  tunnel: [w321 w330] -> w307
                  tunnel: w309 -> [w319 w331]
                  tunnel: w310 -> [w315 _]
                  tunnel: w311 -> [w314 _]
                  tunnel: w308 -> [_ w332]
                  frame False {
                    n162 = call "Master Setup Open.vi"("Master Setup File (in)"=w315) -> ("File Paths (out)"=w318:path[], "Master Setup File (out)"=w322:path)  [unwired: 9 in]
                    n163 = call "Save to History List.vi"("Write to History File"=TRUE, "File pattern label"=w314, "File Path In"=w315) -> ("error out"=w316:errorcluster)  [unwired: 5 in, 3 out]
                    n164 = for {
                      tunnel: [w327] -> w320
                      tunnel: w318 -> [w326] mode=indexing
                      i -> [w328]
                      n165 = call "Master Setup Read Write Setup Paths.vi"("Read (F)/Write (T)"=TRUE, "Pattern Label"=w328, "Master Setup File Path (in)"=w326) -> ("error out"=w327:errorcluster)  [unwired: 4 in, 4 out]
                    }
                    n166 = Bundle By Name(cluster=w319, "Master Setup Path"=w322, "First Run"=FALSE) -> (w321:T8)
                    n167 = call <vilib>:"Clear Errors.vi"("error in (no error)"=w316) -> ()  [unwired: 5 in, 2 out]
                    n168 = case shown="No Error" w320 {
                      frame No Error {
                        n169 = control-ref of="Master Setup File List"() -> (w325:refnum<vi>)
                        n170 = control-ref of="Progress"() -> (w324:refnum<vi>)
                        n171 = call "Master Setup Update Status.vi"("Function"=T12."Get Master Open Status", "Progress Bar Refnum"=w324, "Master Setup List Refnum"=w325) -> ()  [unwired: 5 in]
                      }
                      frame Error {
                      }
                    }
                  }
                  frame True {
                    n172 = case "First Run?" shown="True" w332 {
                      tunnel: w331 -> [w333 w335]
                      tunnel: [w333 w334] -> w330
                      frame False {
                      }
                      frame True {
                        n173 = disable-structure shown="Disabled" {
                          disable-tunnel: w335 -> [_ w341]
                          disable-tunnel: [_ w339] -> w334
                          frame Disabled {
                            # "This case was added so that on first startup, if the operator clicks on cancel, it will trigger all the subpanels to run.  If this case is not added, then all subpanels will have to wait until the operator performs a master open."
                            n174 = flat-sequence {
                              frame #0 {
                                n175 = shared-variable ".\\PC Variables.lvlib\\Master Open"(TRUE ("Master Open")) -> ()  [unwired: 1 in, 1 out]
                              }
                              frame #1 {
                                n176 = Wait (ms)(milliseconds to wait=u32 1000) -> ()  [unwired: 1 out]
                              }
                              frame #2 {
                                n177 = shared-variable ".\\PC Variables.lvlib\\Master Open"(FALSE ("Master Open")) -> ()  [unwired: 1 in, 1 out]
                              }
                            }
                          }
                          frame Enabled {
                            w346 = "Main screen events queue" ("name (unnamed)")
                            # "Skipping the Save Prompt and Exiting the REPS if \nthe user cancels the initial Open Recent dialog."
                            n178 = Bundle By Name(cluster=w341, "Skip Save Prompt?"=TRUE) -> (w339:T8)
                            n179 = Obtain Queue(name (unnamed)=w346, element data type=w346, create if not found? (T)=FALSE) -> (queue out=w344:refnum<queue>, error out=w343:errorcluster)  [unwired: 2 in, 1 out]
                            n180 = Enqueue Element(queue=w344, element="Exit", error in (no error)=w343) -> ()  [unwired: 1 in, 3 out]
                          }
                        }
                      }
                    }
                  }
                }
                n181 = Enqueue Element(queue=w303, element=Master_Setup_States_Enum."Update Display") -> (queue out=w304:refnum<queue>)  [unwired: 2 in, 2 out]
              }
              frame True {
                # "If browse option is selected in the open recent dialog box, then recall the this state again \nwith \"Shortcut Open=False\""
                n182 = Bundle By Name(cluster=w349, "Shortcut Open (From Button)"=FALSE) -> (w348:T7)
                n183 = Enqueue Element(queue=w351, element=Master_Setup_States_Enum."Master Open") -> (queue out=w350:refnum<queue>)  [unwired: 2 in, 2 out]
              }
            }
          }
          frame Enabled {
            w374 = TRUE  # Reset?
            w375 = T21 0 items=["Channel Setup (0)", "PID Setup (1)", "Filter Setup (2)", "CAN Message Setup (3)", "CAN 1 Setup (4)", "CAN 2 Setup (5)", "Digital Inputs Setup (6)", "Digital Outputs Setup (7)", "Logging 1 Setup (8)", "Logging 2 Setup (9)", "Logging 3 Setup (10)", "Setpoint Setup (11)", "Test Series Setup (12)", "Graph Setup (13)", "System Configure (14)", "Header (15)", "Profile Manager (16)", "Post-Mortem Logging (17)", "High-Speed Data (18)", "Statistic Channel Setup (19)", "Ramp Channel Setup (20)", "ETAS INCA Channel Setup (21)", "ETC ECCS Transducer Setup (22)", "ETC ECCS Test Setup (23)", "AVL AK Smoke Meter Setup (24)", "Triggers Setup (25)", "Alarm Limits Setup (26)", "YKWT1 Measurement (27)", "YKWT1 Instrument (28)", "Auto File Settings (29)", "Playback File Setting (30)", "UUT Constants (31)", "UPS Setup (32)", "Differential Channel Setup (33)", "Integral Channel Setup (34)", "Signal Channel Setup (35)", "Calibration Setup (36)", "BNC Setup (37)", "ASAP3 Setup (38)", "Chassis Force Calculations (39)", "Chassis Teststand Losses (40)", "Chassis Vehicle Losses (41)", "Formula Channels (42)", "ASAP3 Map Coords Setup (43)", "Digital Controls Setup (44)", "Push Buttons Setup (45)", "Sliders Setup (46)", "Analog Inline Filter Setup (47)", "Email Setup (48)", "Timer Setup (49)", "Unit Conversion Setup (50)", "Visible Channels (51)", "Main Display Setup (52)", "Message Display Setup (53)", "Input Display Setup (54)", "Unico Parameter Downloads (55)", "Flow Meter Setup (56)", "Channel Zero Offset (57)", "YKWT2 Measurement (58)", "YKWT2 Instrument (59)", "CAN 3 Setup (60)", "CAS Setup (61)", "Accumulation Channel Setup (62)", "Valvetrain Dynamics Setup (63)", "CCP Setup (64)", "System Log Setup (65)", "Throttle Controller (66)"] ("Pattern Label")
            n184 = Unbundle By Name(w378) -> ("Shortcut Open (From Button)"=w380:bool)
            n185 = call "Master Setup File Fault Check.vi"("Reset?"=w374, "Clear File Load Error Ref."=refnum<vi> refnum, "Pattern Label"=w375) -> ("error out"=w373:errorcluster)  [unwired: 11 in, 1 out]
            n186 = call <vilib>:"Clear Errors.vi"("error in (no error)"=w373) -> ()  [unwired: 5 in, 2 out]
            n187 = Select(t=Master_Setup_States_Enum."Open Recent Dialog" ("element"), s=w380, f=Master_Setup_States_Enum."Open Normal Dialog" ("element")) -> (s? t:f=w381:T6)
            n188 = Enqueue Element(queue=w384, element=w381) -> (queue out=w383:refnum<queue>)  [unwired: 2 in, 2 out]
          }
        }
      }
      frame "Open Recent Dialog" {
        n189 = Unbundle By Name(w393) -> ("First Run"=w390:bool, "Master Pattern Label"=w394:string)
        n190 = Select(t="Exit REPS" ("Cancel Button String"), s=w390, f="") -> (s? t:f=w397:string)
        n191 = call "Prompt for Recent Files.vi"("File pattern label"=w394, "Cancel Button String"=w397) -> ("File to Open"=w386:string, "Cancelled"=w385:bool, "Browse for file"=w387:bool)  [unwired: 1 in]
        n192 = And(x=w390, y=w385) -> (x .and. y?=w391:bool)
        n193 = case "Open Recent dialog cancelled on REPS Startup (i.e., First Run)?" shown="False" w391 {
          tunnel: w393 -> [w402 w434]
          tunnel: [w401 w433] -> w392
          tunnel: w389 -> [w406 w432]
          tunnel: [w405 w432] -> w388
          tunnel: w387 -> [w404 _]
          tunnel: w386 -> [w403 _]
          tunnel: w385 -> [w400 _]
          frame False {
            n194 = case "Browse Button clicked in the dialog?" shown="False" w404 {
              tunnel: w406 -> [w412 w425]
              tunnel: [w411 w424] -> w405
              tunnel: w403 -> [w410 _]
              tunnel: w402 -> [w409 w422]
              tunnel: [w408 w422] -> w401
              tunnel: w400 -> [w407 _]
              frame False {
                n195 = case "Open Recent dialog Cancelled?" shown="False" w407 {
                  tunnel: w412 -> [w418 w420]
                  tunnel: [w417 w420] -> w411
                  tunnel: w410 -> [w415 _]
                  tunnel: w409 -> [w414 w421]
                  tunnel: [w413 w421] -> w408
                  frame False {
                    # "It's assumed that OK button is clicked if both browse and cancel buttons are\nnot clicked.  Then call \"Open Selected Master File\""
                    n196 = String To Path(string=w415) -> (path=w416:path)
                    n197 = Bundle By Name(cluster=w414, "Master Setup Path"=w416) -> (w413:T8)
                    n198 = Enqueue Element(queue=w418, element=Master_Setup_States_Enum."Open Selected Master File") -> (queue out=w417:refnum<queue>)  [unwired: 2 in, 2 out]
                  }
                  frame True {
                    # "Do nothing if the Open Recent dialog is cancelled"
                  }
                }
              }
              frame True {
                # "Open normal file dialog if Browse button is clicked."
                n199 = Enqueue Element(queue=w425, element=Master_Setup_States_Enum."Open Normal Dialog") -> (queue out=w424:refnum<queue>)  [unwired: 2 in, 2 out]
              }
            }
          }
          frame True {
            w431 = "Main screen events queue" ("name (unnamed)")
            # "Skipping the Save Prompt and Exiting the REPS if \nthe user cancels the initial Open Recent dialog."
            n200 = Bundle By Name(cluster=w434, "Skip Save Prompt?"=TRUE) -> (w433:T8)
            n201 = Obtain Queue(name (unnamed)=w431, element data type=w431, create if not found? (T)=FALSE) -> (queue out=w429:refnum<queue>, error out=w428:errorcluster)  [unwired: 2 in, 1 out]
            n202 = Enqueue Element(queue=w429, element="Exit", error in (no error)=w428) -> ()  [unwired: 1 in, 3 out]
          }
        }
      }
      frame "Open Normal Dialog" {
        n203 = Unbundle By Name(w443) -> ("Shortcut Open (From Button)"=w436:bool)
        n204 = Unbundle By Name(w439) -> ("Master Setup Path"=w447:path, "Master Pattern"=w445:string, "Master Pattern Label"=w449:string)
        n205 = Strip Path(path=w447) -> (stripped path=w448:path)  [unwired: 1 out]
        n206 = call "File Dialog3"("start path"=w448, "prompt"="Please Select a Master Setup File to Open...", "pattern (all files)"=w445, "pattern label"=w449) -> ("selected path"=w440:path, "cancelled"=w437:bool, "error out"=w444:errorcluster)  [unwired: 8 in, 1 out]
        n207 = And(x=w436, y=w437) -> (x .and. y?=w435:bool)
        n208 = call <vilib>:"Clear Errors.vi"("error in (no error)"=w444) -> ()  [unwired: 5 in, 2 out]
        n209 = case "Normal file dialog opened from Open Recent Dialog but cancelled?" shown="False" w435 {
          tunnel: w437 -> [w456 _]
          tunnel: w442 -> [w455 w468]
          tunnel: [w454 w467] -> w441
          tunnel: w440 -> [w453 _]
          tunnel: w439 -> [w452 w465]
          tunnel: [w451 w465] -> w438
          frame False {
            n210 = case shown="False" w456 {
              tunnel: w455 -> [w462 w464]
              tunnel: [w461 w464] -> w454
              tunnel: w453 -> [w459 _]
              tunnel: w452 -> [w458 w463]
              tunnel: [w457 w463] -> w451
              frame False {
                # "User has selected some file to open."
                n211 = Bundle By Name(cluster=w458, "Master Setup Path"=w459) -> (w457:T8)
                n212 = Enqueue Element(queue=w462, element=Master_Setup_States_Enum."Open Selected Master File") -> (queue out=w461:refnum<queue>)  [unwired: 2 in, 2 out]
              }
              frame True {
                # "If user cancelled the normal dialog button and this state is \ntriggered from normal Master Open, then Do Nothing"
              }
            }
          }
          frame True {
            # "Open recent dialog again if this normal dialog is opened\nfrom \"Browse\" button of the Open Recent dialog but cancelled"
            n213 = Enqueue Element(queue=w468, element=Master_Setup_States_Enum."Open Recent Dialog") -> (queue out=w467:refnum<queue>)  [unwired: 2 in, 2 out]
          }
        }
      }
      frame "Open Selected Master File" {
        n214 = Unbundle By Name(w471) -> ("Master Pattern Label"=w470:string, "Master Setup Path"=w469:path)
        n215 = local write "File Path"(w469) -> ()
        n216 = call "Master Setup Open.vi"("Master Setup File (in)"=w469) -> ("File Paths (out)"=w474:path[])  [unwired: 9 in, 1 out]
        n217 = call "Save to History List.vi"("Write to History File"=TRUE, "File pattern label"=w470, "File Path In"=w469) -> ("error out"=w476:errorcluster)  [unwired: 5 in, 3 out]
        n218 = for {
          tunnel: [w485] -> w473
          tunnel: w474 -> [w484] mode=indexing
          i -> [w486]
          n219 = call "Master Setup Read Write Setup Paths.vi"("Read (F)/Write (T)"=TRUE, "Pattern Label"=w486, "Master Setup File Path (in)"=w484) -> ("error out"=w485:errorcluster)  [unwired: 4 in, 4 out]
        }
        n220 = Bundle By Name(cluster=w471, "First Run"=FALSE) -> (w472:T8)
        n221 = call <vilib>:"Clear Errors.vi"("error in (no error)"=w476) -> ()  [unwired: 5 in, 2 out]
        n222 = case shown="No Error" w473 {
          frame No Error {
            n223 = control-ref of="Master Setup File List"() -> (w483:refnum<vi>)
            n224 = control-ref of="Progress"() -> (w482:refnum<vi>)
            n225 = call "Master Setup Update Status.vi"("Function"=T12."Get Master Open Status", "Progress Bar Refnum"=w482, "Master Setup List Refnum"=w483) -> ()  [unwired: 5 in]
          }
          frame Error {
          }
        }
      }
      frame "WINZIP Export" {
        n226 = Unbundle By Name(w494) -> ("Sorted Titles Indices"=w493:i32[], "Sorted Titles"=w491:string[], "Master Setup Path"=w488:path)
        n227 = for {
          tunnel: w489 -> [w499]
          tunnel: w493 -> [w498] mode=indexing
          tunnel: [w497] -> w492 mode=indexing
          n228 = Index Array(array=w499, index=w498) -> (element=w497:path)
        }
        n229 = call "Master Setup Export.vi"("Master Setup Path"=w488, "Setup Files"=w491, "Setup File Paths"=w492) -> ()  [unwired: 9 in]
      }
      frame "WINZIP Import" {
        n230 = Unbundle By Name(w509) -> ("Master Setup Path"=w507:path, "Sorted Titles"=w503:string[], "Sorted Titles Indices"=w501:i32[])
        n231 = call "Master Setup Import.vi"("Sorted Titles Indices"=w501, "Sorted Titles"=w503, "Master Setup Path In"=w507, "Master Setup In"=w500) -> ("Cancelled"=w504:bool, "Master Setup Path Out"=w506:path, "Master Setup Out"=w510:path[])  [unwired: 5 in]
        n232 = case shown="False" w504 {
          tunnel: w511 -> [w516 w528]
          tunnel: w510 -> [w513 _]
          tunnel: w509 -> [w520 w529]
          tunnel: [w519 w529] -> w508
          tunnel: w506 -> [w518 _]
          tunnel: [w517 w528] -> w505
          frame False {
            n233 = Bundle By Name(cluster=w520, "Master Setup Path"=w518) -> (w519:T8)
            n234 = for {
              tunnel: [w522] -> w515
              tunnel: w513 -> [w521] mode=indexing
              i -> [w523]
              n235 = call "Master Setup Read Write Setup Paths.vi"("Read (F)/Write (T)"=TRUE, "Pattern Label"=w523, "Master Setup File Path (in)"=w521) -> ("error out"=w522:errorcluster)  [unwired: 4 in, 4 out]
            }
            n236 = case shown="No Error" w515 {
              frame No Error {
                n237 = control-ref of="Master Setup File List"() -> (w527:refnum<vi>)
                n238 = control-ref of="Progress"() -> (w526:refnum<vi>)
                n239 = call "Master Setup Update Status.vi"("Function"=T12."Get Master Open Status", "Progress Bar Refnum"=w526, "Master Setup List Refnum"=w527) -> ()  [unwired: 5 in]
              }
              frame Error {
              }
            }
            n240 = Enqueue Element(queue=w516, element=Master_Setup_States_Enum."Update Display") -> (queue out=w517:refnum<queue>)  [unwired: 2 in, 2 out]
          }
          frame True {
            # "Cancelled"
          }
        }
      }
      frame "WINZIP Auto Backup" {
        w544 = TRUE  # Export all files?
        n241 = Unbundle By Name(w533) -> ("Sorted Titles Indices"=w534:i32[], "Sorted Titles"=w536:string[], "Master Setup Path"=w545:path)
        n242 = for {
          tunnel: w532 -> [w552]
          tunnel: w534 -> [w551] mode=indexing
          tunnel: [w550] -> w535 mode=indexing
          n243 = Index Array(array=w552, index=w551) -> (element=w550:path)
        }
        n244 = shared-variable ".\\PC Variables Master.lvlib\\Master Auto Backup"(FALSE ("Master Auto Backup")) -> ()  [unwired: 1 in, 1 out]
        n245 = Format Date/Time String(time format string (%c)="%y%m%d %H%M%S") -> (date/time string=w539:string)  [unwired: 2 in]
        n246 = call <vilib>:"Get File Extension.vi"("file"=w545) -> ("filename without extension"=w546:string)  [unwired: 6 in, 4 out]
        n247 = call "Check if Path OK.vi"("Create if not found? (F)"=TRUE, "Path"=w531) -> ("Path"=w541:path)  [unwired: 7 in, 2 out]
        n248 = Format Into String(format string="%s %s.zip", w539, w546) -> (resulting string=w542:string)  [unwired: 2 in, 1 out]
        n249 = Build Path(base path=w541, name or relative path=w542) -> (appended path=w543:path)
        n250 = call "Master Setup Export.vi"("Export all files?"=w544, "Zip File Path"=w543, "Master Setup Path"=w545, "Setup Files"=w536, "Setup File Paths"=w535) -> ()  [unwired: 7 in]
      }
      frame "Exit" {
      }
    }
  }
  n251 = control-ref of="Master Exit"() -> (w28:refnum<vi>)
  n252 = control-ref of="Master Open"() -> (w29:refnum<vi>)
  n253 = control-ref of="Master Save"() -> (w30:refnum<vi>)
  n254 = vi-ref "Event Log Subpanel.vi"() -> (w16:refnum<vi>)
  n255 = call "Front Panel Show-Hide Menu and Tool Bars.vi"("Current VI Path"=w22) -> ()  [unwired: 1 out]
  n256 = invoke class="VI" method="Run VI"(reference=w16, "Wait until done"=FALSE ("Wait Until Done"), "Auto Dispose Ref"=TRUE ("Auto Dispose Reference")) -> (reference out=w19:refnum<vi>, error out=w20:errorcluster)  [unwired: 2 in, 3 out]
  n257 = invoke on="Event Log" class="SubPanel" method="Insert VI"("VI Ref"=w16) -> ()  [unwired: 3 in, 4 out]
  n258 = call "Master Setup Read Write References.vi"("Master Exited (in)"=w28, "Read (F)/ Write (T)"=TRUE, "Master Open (in)"=w29, "Master Save (in)"=w30) -> ()  [unwired: 6 in, 6 out]
  n259 = Close Reference(reference=w19, error in (no error)=w20) -> (error out=w21:errorcluster)
  n260 = call <vilib>:"Clear Errors.vi"("error in (no error)"=w21) -> ()  [unwired: 5 in, 2 out]
  n261 = while {
    stop <- w585 stop-if-true
    w567 = T6[] [enum."WINZIP Auto Backup", enum."Update Display", enum."Prompt to Save", enum."Exit"] items=["Initialize", "Update Display", "Poll", "Prompt to Save", "Master Save", "Master Open", "Open Recent Dialog", "Open Normal Dialog", "Open Selected Master File", "WINZIP Export", "WINZIP Import", "WINZIP Auto Backup", "Exit"] ("States to Add to Queue")
    # "Show/Hide the debug tab."
    n262 = shared-variable ".\\PC Variables Master.lvlib\\Master Update Display"() -> (w560:bool)  [unwired: 1 in, 1 out]
    n263 = shared-variable ".\\PC Variables Master.lvlib\\Master Auto Backup"() -> (w559:bool)  [unwired: 1 in, 1 out]
    n264 = Wait (ms)(milliseconds to wait=u32 100) -> ()  [unwired: 1 out]
    n265 = shared-variable ".\\PC Variables.lvlib\\Master Exited"() -> (w562:bool)  [unwired: 1 in, 1 out]
    n266 = shared-variable ".\\PC Variables.lvlib\\Master Open"() -> (w563:bool)  [unwired: 1 in, 1 out]
    n267 = shared-variable ".\\PC Variables.lvlib\\Master Save"() -> (w564:bool)  [unwired: 1 in, 1 out]
    n268 = shared-variable ".\\PC Variables.lvlib\\REPS Exited"() -> (w558:bool)  [unwired: 1 in, 1 out]
    n269 = shared-variable ".\\PC Variables.lvlib\\Login User"() -> (w561:string)  [unwired: 1 in, 1 out]
    "Login User" <- w561
    n270 = property on="RT Update Error" class="Arr (strict)"() -> ("Index Values"=w581:u32[])  [unwired: 2 in, 2 out]
    n271 = Build Array(w559, w560, w558, w558) -> (w568:bool[])
    n272 = feedback-in #2(w563) -> ()
    n273 = feedback #2() -> (w575:bool)  [unwired: 1 in]
    n274 = feedback-in #3(w564) -> ()
    n275 = feedback #3() -> (w574:bool)  [unwired: 1 in]
    n276 = feedback-in #4(w561) -> ()
    n277 = feedback #4() -> (w570:string)  [unwired: 1 in]
    n278 = feedback-in #5(w581) -> ()
    n279 = feedback #5() -> (w582:u32[])  [unwired: 1 in]
    n280 = feedback-in #6(w560) -> ()
    n281 = feedback #6() -> (w576:bool)  [unwired: 1 in]
    n282 = Not Equal?(x=w560, y=w576) -> (x != y?=w577:bool)
    n283 = Not Equal?(x=w563, y=w575) -> (x != y?=w579:bool)
    n284 = Not Equal?(x=w564, y=w574) -> (x != y?=w578:bool)
    n285 = feedback-in #7(w568) -> ()
    n286 = feedback #7() -> (w569:bool[])  [unwired: 1 in]
    n287 = Equal?(x=w561, y="Administrator" ("Login User")) -> (x = y?=w571:bool)
    n288 = Not Equal?(x=w561, y=w570) -> (x != y?=w572:bool)
    n289 = Not Equal?(x=w581, y=w582) -> (x != y?=w583:bool)
    n290 = Greater?(x=w568, y=w569) -> (0:w566:bool[])
    n291 = case shown="True" w572 {
      tunnel: w571 -> [_ w594]
      frame False {
      }
      frame True {
        n292 = property on="Tab Control" class="TabCtl (strict)"("Tabs Visible?"=w594, "Value"=T2."Master Setup List" ("Tab Control")) -> ()  [unwired: 2 in, 2 out]
      }
    }
    n293 = case shown="True" w583 {
      tunnel: w581 -> [_ w595]
      frame False {
      }
      frame True {
        n294 = property on="Master Setup Titles" class="Arr (strict)"("Index Values"=w595) -> ()  [unwired: 2 in, 2 out]
        n295 = property on="Master Open Status" class="Arr (strict)"("Index Values"=w595) -> ()  [unwired: 2 in, 2 out]
        n296 = property on="Master Save Status" class="Arr (strict)"("Index Values"=w595) -> ()  [unwired: 2 in, 2 out]
        n297 = property on="File Error" class="Arr (strict)"("Index Values"=w595) -> ()  [unwired: 2 in, 2 out]
        n298 = property on="Convert Error" class="Arr (strict)"("Index Values"=w595) -> ()  [unwired: 2 in, 2 out]
        n299 = property on="RT Update Error" class="Arr (strict)"("Index Values"=w595) -> ()  [unwired: 2 in, 2 out]
      }
    }
    n300 = Compound Arithmetic op=OR("Refresh", w579, w578, w577) -> (w580:bool)
    n301 = Or Array Elements(Boolean array=w566) -> (logical OR=w565:bool)
    n302 = case shown="True" w562 {
      selector: w562 -> [_ w601]
      tunnel: [_ w601] -> w585
      frame False {
      }
      frame True {
        n303 = property on="Master Exit" class="Bool (strict)"("Val(Sgnl)"=w601) -> ()  [unwired: 2 in, 2 out]
      }
    }
    n304 = case shown="True" w580 {
      frame False {
      }
      frame True {
        n305 = call "Master Setup Check If Master Open Completed.vi"() -> ("Master Open Status"=→"Master Open Status":bool[])  [unwired: 7 in, 4 out]
        n306 = call "Master Setup Check If Master Save Completed.vi"() -> ("Master Save Status"=→"Master Save Status":bool[])  [unwired: 7 in, 4 out]
        n307 = call "Master Setup Read Write File Errors.vi"() -> ("File Error (out)"=→"File Error":bool[])  [unwired: 10 in, 1 out]
        n308 = call "Master Setup Read Write Convert Errors.vi"() -> ("Convert Error (out)"=→"Convert Error":bool[])  [unwired: 10 in, 1 out]
        n309 = call "Master Setup Read Write RT Update Errors.vi"() -> ("Real-Time Update Status (out)"=→"RT Update Error":bool[])  [unwired: 9 in, 2 out]
      }
    }
    n310 = case shown="True" w579 {
      tunnel: w563 -> [_ w603]
      frame False {
      }
      frame True {
        n311 = property on="Master Open" class="Bool (strict)"("Val(Sgnl)"=w603) -> ()  [unwired: 2 in, 2 out]
        "Master Open Indicator" <- w603
      }
    }
    n312 = case shown="True" w578 {
      tunnel: w564 -> [_ w602]
      frame False {
      }
      frame True {
        n313 = property on="Master Save" class="Bool (strict)"("Val(Sgnl)"=w602) -> ()  [unwired: 2 in, 2 out]
        "Master Save Indicator" <- w602
      }
    }
    n314 = case shown="True" w565 {
      tunnel: w566 -> [_ w591]
      tunnel: w567 -> [_ w589]
      frame False {
      }
      frame True {
        n315 = Not(x=w591) -> (.not. x?=w590:bool[])
        n316 = call "Delete items from array (U16).vi"("Items to delete"=w590, "Array"=w589) -> ("Array with items deleted"=w588:u16[])  [unwired: 9 in]
        n317 = call "Timeout State Queuer.vi"("Action"=T10."Write U16 Queue", "States to Queue (U16)"=w588, "Name of queue"="Master Setup") -> ()  [unwired: 7 in, 2 out]
      }
    }
  }
  n318 = Flush Queue(queue=w32) -> (queue out=w34:refnum<queue>, error out=w33:errorcluster)  [unwired: 1 in, 1 out]
  n319 = Release Queue(queue=w26, force destroy? (F)=FALSE) -> ()  [unwired: 1 in, 3 out]
  n320 = shared-variable ".\\PC Variables.lvlib\\Master Exited"(w1) -> ()  [unwired: 1 in, 1 out]
  n321 = shared-variable ".\\PC Variables.lvlib\\Master Exited"(FALSE ("Master Exited")) -> ()  [unwired: 1 in, 1 out]
  n322 = Release Queue(queue=w34, error in (no error)=w33) -> (error out=w4:errorcluster)  [unwired: 1 in, 2 out]
  n323 = Close Reference(reference=w3, error in (no error)=w4) -> ()  [unwired: 1 out]
